vi "Open Untitled VI__ogtk.vi"(5 "Open Front Panel? (TRUE)":bool=TRUE, 6 "Return Refnum? (FALSE)":bool) -> (1 "error out":errorcluster, 2 "VI Refnum":refnum<vi>)   [LabVIEW 2009]
doc: "Creates and opens a new Untitled VI. A reference to the newly created VI will be returned if a TRUE is wired to the \"Return Refnum\", otherwise \"Not a Refnum\" is returned. The front panel of the newly create VI will be opened unless a FALSE is wired to the \"Open Front Panel\" input."
panel:
  # "Open Untitled VI.vi\n\nCreates and opens a new Untitled VI the VI calling this function.\n\nPlease visit http://www.OpenG.org to learn about the\nOpen Source LabVIEW software movement.\n\nNOTICE -- YOU MUST LEAVE THIS NOTICE IN PLACE.  PER THE TERMS OF THE LICENSE BELOW, YOU MAY SUBLICENSE THIS SOFTWARE \nIN ANY WAY THAT DOES NOT CONFLICT WITH THIS LICENSE.\n\n### BSD License (http://www.opensource.org/licenses/bsd-license.php) Begin ###\n \nCopyright (c) 2002, Jim Kring <jim@jimkring.com>\n\nAll rights reserved.\n\nRedistribution and use in source and binary forms, with or without modification, are permitted provided that the following conditions are met:\n\n    * Redistributions of source code must retain the above copyright notice, this list of conditions and the following disclaimer.\n    * Redistributions in binary form must reproduce the above copyright notice, this list of conditions and the following disclaimer in the \n       documentation and/or other materials provided with the distribution.\n    * Neither the name of SciWare, James Kring, Inc., nor the names of its contributors may be used to endorse or promote products derived \n       from this software without specific prior written permission.\n\nTHIS SOFTWARE IS PROVIDED BY THE COPYRIGHT HOLDERS AND CONTRIBUTORS \"AS IS\" AND ANY EXPRESS OR IMPLIED WARRANTIES, \nINCLUDING, BUT NOT LIMITED TO, THE IMPLIED WARRANTIES OF MERCHANTABILITY AND FITNESS FOR A PARTICULAR PURPOSE ARE \nDISCLAIMED. IN NO EVENT SHALL THE COPYRIGHT OWNER OR CONTRIBUTORS BE LIABLE FOR ANY DIRECT, INDIRECT, INCIDENTAL,\n SPECIAL, EXEMPLARY, OR CONSEQUENTIAL DAMAGES (INCLUDING, BUT NOT LIMITED TO, PROCUREMENT OF SUBSTITUTE GOODS OR \nSERVICES; LOSS OF USE, DATA, OR PROFITS; OR BUSINESS INTERRUPTION) HOWEVER CAUSED AND ON ANY THEORY OF LIABILITY, \nWHETHER IN CONTRACT, STRICT LIABILITY, OR TORT (INCLUDING NEGLIGENCE OR OTHERWISE) ARISING IN ANY WAY OUT OF THE USE \nOF THIS SOFTWARE, EVEN IF ADVISED OF THE POSSIBILITY OF SUCH DAMAGE.\n\n### BSD License End ###"
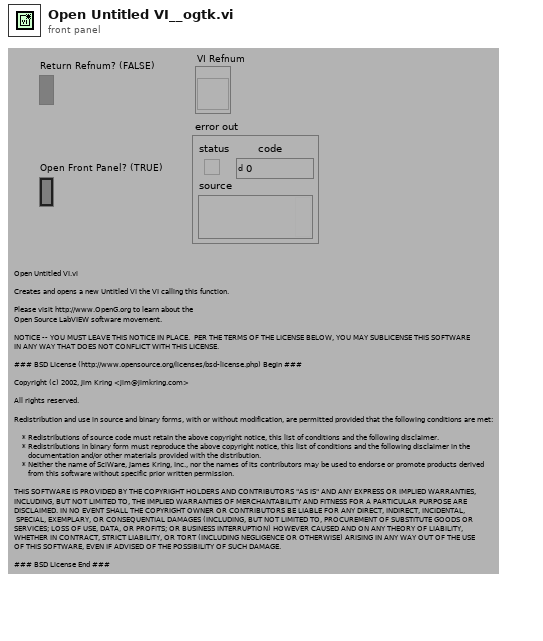
[diagram p1: front panel]
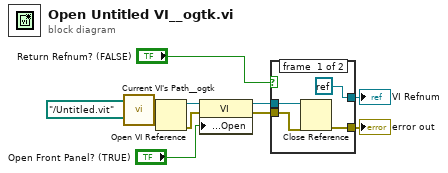
[diagram p0: block diagram]
diagram:
  n1 = call <userlib>:"Current VI's Path__ogtk.vi"("Relative path (.)"=path "../Untitled.vit") -> ("Current VI's Path (+ Relative)"=w1:path)
  n2 = Open VI Reference(vi path=w1) -> (vi reference=w10:refnum<vi>, error out=w8:errorcluster)  [unwired: 5 in]
  n3 = property class="VI"(reference=w10, error in=w8, "Front Panel Window:Open"="Open Front Panel? (TRUE)") -> (reference out=w9:refnum<vi>, error out=w7:errorcluster)
  n4 = case shown="False" "Return Refnum? (FALSE)" {
    tunnel: w9 -> [w14 w16]
    tunnel: w7 -> [w13 w15]
    tunnel: [w12 w15] -> w6
    tunnel: [refnum<k0> refnum w16] -> w4
    frame #0 {
      n5 = Close Reference(reference=w14, error in (no error)=w13) -> (error out=w12:errorcluster)
    }
    frame #1 {
    }
  }
  "error out" <- w6
  "VI Refnum" <- w4
